vi "PH_Revolver-GUI_6P.ProcCases.vi"(0 "i ref in":refnum<vi>, 1 "selector":string, 2 "data":i8[](array[numeric]), 3 "call cluster":T1={"Object"="", "Selector"="", "CallType"=enum."synchronous", "Async Object"="", "Async Selector"="", "Data Descriptor"="", "Data"=[], "Error #"=0, "Expire"=0}, 5 "error in":errorcluster) -> (14 "i ref out":refnum<vi>, 17 "answer cluster":T1={"Object"="", "Selector"="", "CallType"=enum."synchronous", "Async Object"="", "Async Selector"="", "Data Descriptor"="", "Data"=[], "Error #"=0, "Expire"=0}, 19 "error out":errorcluster)   [LabVIEW 2014, in "PH_Revolver-GUI_6P.lvlib"]
doc: "This method is called by a process from within the default case in the event loop. The methods of a class that are linked to events will be called from THIS method. Add your code here."
uses:
  PH_Revolver-GUI_6P.lvlib
  CS_Core/CSSystem/CoreDefs/CoreDefs.call_type.ctl
  CS_Core/BaseProcess/BaseProcess.descriptor string definition.ctl
  CS_Core/CSSystem/CoreDefs/CoreDefs.rawDataType.ctl
  PH_Revolver-GUI_6P.Position.ctl
  CS_Core/CSSystem/CoreLib/CoreLib.string 2 byte array.vi
  CS_Core/CSSystem/CoreLib/CoreLib.byte array 2 short.vi
  CS_Core/BaseProcess/BaseProcess.lvlib
  CS_Core/CSSystem/CoreLib/CoreLib.lvlib
  CS_Core/CAEObj/CAEObj.lvlib
  PH_Basics/PH_PSDBWriter/PH_PSDBWriter.lvlib
  PH_Basics/PH_Stepmotor_BaseClass/PH_Stepmotor_BaseClass.lvlib
  PH_Basics/PH_AxisGUI_BaseClass/PH_AxisGUI_BaseClass.lvlib
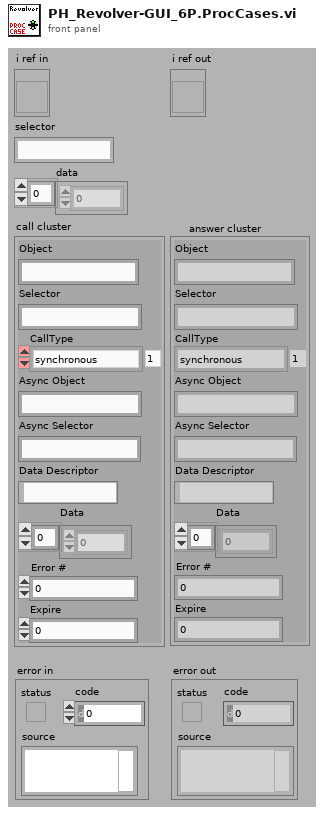
[diagram p1: front panel]
types:
  T1 = typedef "CoreDefs.call_type.ctl" = cluster{"Object":string, "Selector":string, "CallType":enum16{"simple", "synchronous", "asynchronous"}, "Async Object":string, "Async Selector":string, "Data Descriptor":T2, "Data":T3, "Error #":i32, "Expire":u32}
  T2 = typedef "BaseProcess.lvlib/BaseProcess.descriptor string definition.ctl" = string
  T3 = typedef "CoreDefs.rawDataType.ctl" = i8[]
  T4 = typedef "PH_PSDBWriter.lvlib/PH_PSDBWriter.PHELIX-Subsystems.ctl" = i32
  T5 = typedef "PH_Stepmotor_BaseClass.lvlib/PH_Stepmotor_BaseClass.Axis Information.ctl" = cluster{"Scaled Position":dbl, "Activity":T6}
  T6 = typedef "PH_Stepmotor_BaseClass.lvlib/PH_Stepmotor_BaseClass.Axis Activity.ctl" = enum16{"No Information", "stopped", "running", "Failure", "Alarm", "stopped at backward ES", "stopped at foreward ES"}
  T7 = typedef "PH_Revolver-GUI_6P.lvlib/PH_Revolver-GUI_6P.Position.ctl" = u16
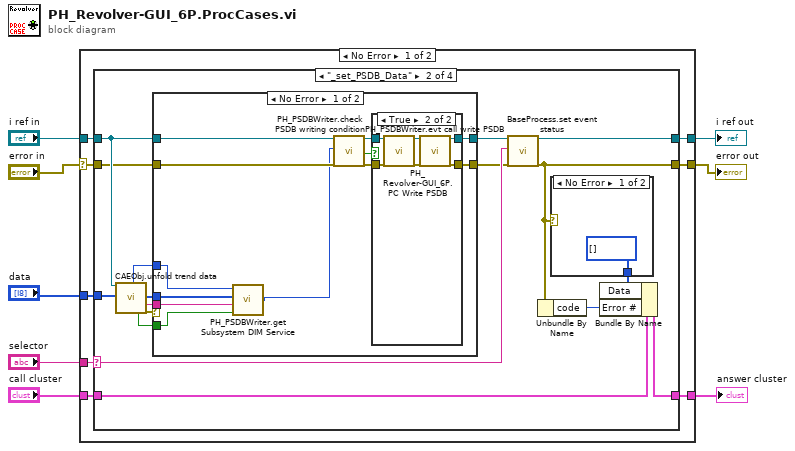
[diagram p0: block diagram]
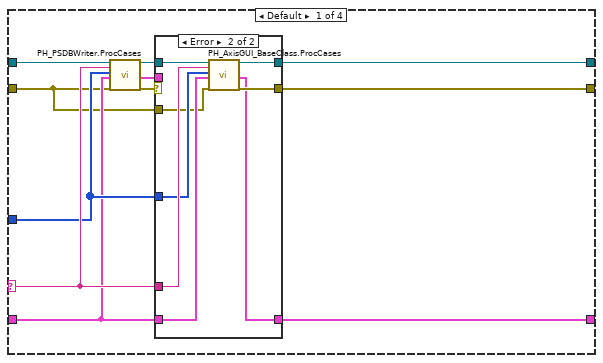
[diagram p2: hidden frame]
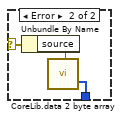
[diagram p6: hidden frame]
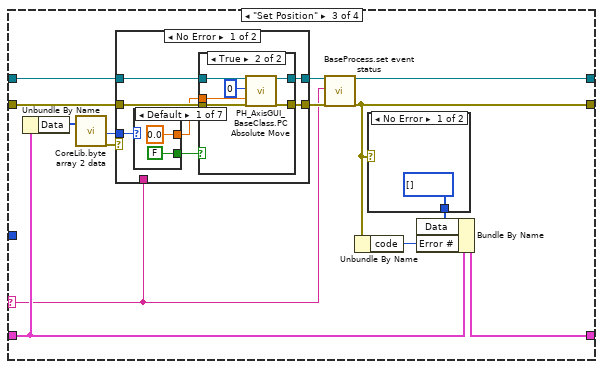
[diagram p7: hidden frame]
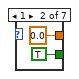
[diagram p9: hidden frame]
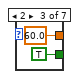
[diagram p10: hidden frame]
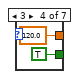
[diagram p11: hidden frame]
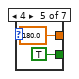
[diagram p12: hidden frame]
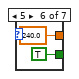
[diagram p13: hidden frame]
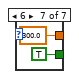
[diagram p14: hidden frame]
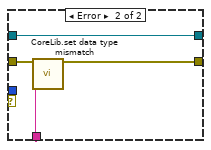
[diagram p15: hidden frame]
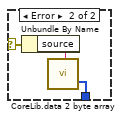
[diagram p16: hidden frame]
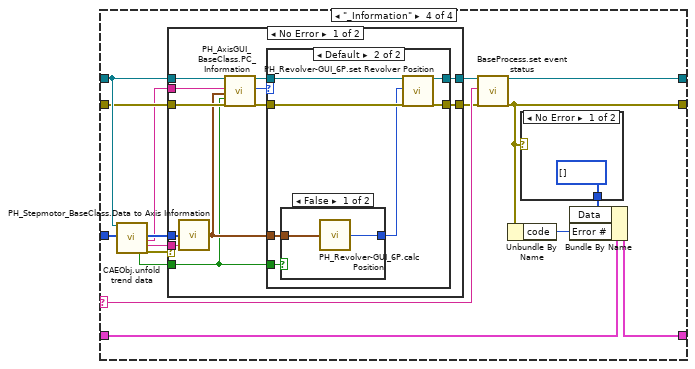
[diagram p17: hidden frame]
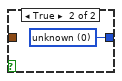
[diagram p19: hidden frame]
diagram:
  n1 = case shown="No Error" "error in" {
    selector: "error in" -> [w9 w181]
    tunnel: "selector" -> [w16 _]
    tunnel: [w15 w180] -> w7
    tunnel: "call cluster" -> [w14 w180]
    tunnel: "i ref in" -> [w13 w182]
    tunnel: [w12 w182] -> w4
    tunnel: [w11 w181] -> w3
    tunnel: "data" -> [w10 _]
    frame No Error {
      n2 = case shown="\"_set_PSDB_Data\"" w16 {
        selector: w16 -> [w22 w49 w82 w146]
        tunnel: w13 -> [w27 w43 w87 w138]
        tunnel: [w24 w52 w93 w145] -> w12
        tunnel: w14 -> [w20 w54 w86 w148]
        tunnel: [w19 w50 w91 w143] -> w15
        tunnel: w9 -> [w17 w40 w85 w136]
        tunnel: [w26 w53 w94 w147] -> w11
        tunnel: w10 -> [w21 w39 _ w134]
        frame Default {
          n3 = call "PH_PSDBWriter.ProcCases.vi"("i ref in"=w27, "selector"=w22, "Data"=w21, "call cluster"=w20, "error in"=w17) -> ("i ref out"=w25:refnum<vi>, "answer cluster"=w18:T1, "error out"=w23:errorcluster)  [unwired: 12 in]
          n4 = case shown="Error" w23 {
            selector: w23 -> [w29 _]
            tunnel: [w29 w38] -> w26
            tunnel: w25 -> [w30 w37]
            tunnel: [w30 w36] -> w24
            tunnel: w22 -> [_ w35]
            tunnel: w21 -> [_ w34]
            tunnel: w20 -> [_ w33]
            tunnel: [w28 w32] -> w19
            tunnel: w18 -> [w28 _]
            tunnel: w17 -> [_ w31]
            frame No Error {
            }
            frame Error {
              n5 = call "PH_AxisGUI_BaseClass.ProcCases.vi"("i ref in"=w37, "selector"=w35, "data"=w34, "call cluster"=w33, "error in"=w31) -> ("i ref out"=w36:refnum<vi>, "answer cluster"=w32:T1, "error out"=w38:errorcluster)  [unwired: 12 in]
            }
          }
        }
        frame "_set_PSDB_Data" {
          n6 = call "CAEObj.unfold trend data.vi"("i ref in"=w43, "raw trend data"=w39) -> ("quality"=w48:i32, "no link"=w45:bool, "data"=w47:i8[], "typeDescriptor"=w46:string, "error out"=w44:errorcluster)  [unwired: 9 in, 4 out]
          n7 = case shown="No Error" w44 {
            tunnel: w40 -> [w67 w77]
            tunnel: [w66 w76] -> w42
            tunnel: [w65 w77] -> w41
            tunnel: w43 -> [w63 w76]
            tunnel: w45 -> [w57 _]
            tunnel: w46 -> [w59 _]
            tunnel: w47 -> [w60 _]
            tunnel: w48 -> [w58 _]
            frame No Error {
              n8 = call "PH_PSDBWriter.get Subsystem DIM Service.vi"("no link"=w57, "typeDescriptor"=w59, "data"=w60, "quality"=w58) -> ("PHELIX Subsystems"=w56:T4)
              n9 = call "PH_PSDBWriter.check PSDB writing condition.vi"("i ref in"=w63, "wanted Subsystem"=w56, "error IO"=w67) -> ("i ref out"=w62:refnum<vi>, "write PSDB?"=w61:bool, "error out"=w64:errorcluster)  [unwired: 14 in]
              n10 = case shown="True" w61 {
                tunnel: w64 -> [w68 w75]
                tunnel: [w69 w72] -> w66
                tunnel: [w68 w70] -> w65
                tunnel: w62 -> [w69 w74]
                frame False {
                }
                frame True {
                  n11 = call "PH_Revolver-GUI_6P.PC Write PSDB.vi"("i ref in"=w74, "error IO"=w75) -> ("i ref out"=w73:refnum<vi>, "error out"=w71:errorcluster)  [unwired: 16 in]
                  n12 = call "PH_PSDBWriter.evt call write PSDB.vi"("i ref in"=w73, "error in (no error)"=w71) -> ("i ref out"=w72:refnum<vi>, "error out"=w70:errorcluster)  [unwired: 16 in]
                }
              }
            }
            frame Error {
            }
          }
          n13 = call "BaseProcess.set event status.vi"("i ref in"=w42, "EventStatus"=w49, "error in (no error)"=w41) -> ("i ref out"=w52:refnum<vi>, "error out"=w53:errorcluster)  [unwired: 14 in, 1 out]
          n14 = Unbundle By Name(w53) -> ("code"=w55:i32)
          n15 = case shown="No Error" w53 {
            selector: w53 -> [_ w81]
            tunnel: [T3 [] ("byteArray out") w79] -> w51
            frame No Error {
            }
            frame Error {
              n16 = Unbundle By Name(w81) -> ("source"=w80:string)
              n17 = call-poly "CoreLib.data 2 byte array.vi"("string"=w80) -> ("byteArray out"=w79:T3)  [unwired: 18 in]
            }
          }
          n18 = Bundle By Name(cluster=w54, "Data"=w51, "Error #"=w55) -> (w50:T1)
        }
        frame "Set Position" {
          n19 = Unbundle By Name(w86) -> ("Data"=w90:T3)
          n20 = call-poly "CoreLib.byte array 2 data.vi"("byteArray"=w90) -> ("i16"=w88:i16, "error out"=w89:errorcluster)  [unwired: 16 in, 1 out]
          n21 = case shown="No Error" w89 {
            tunnel: [w98 w128] -> w84
            tunnel: w87 -> [w99 w128]
            tunnel: w85 -> [w101 w127]
            tunnel: [w100 w126] -> w83
            tunnel: w82 -> [_ w125]
            tunnel: w88 -> [w102 _]
            frame No Error {
              n22 = case shown="Default" w102 {
                tunnel: [0.0 0.0 60.0 120.0 180.0 240.0 300.0] -> w97
                tunnel: [FALSE TRUE TRUE TRUE TRUE TRUE TRUE] -> w96
                frame Default {
                }
                frame 1 {
                }
                frame 2 {
                }
                frame 3 {
                }
                frame 4 {
                }
                frame 5 {
                }
                frame 6 {
                }
              }
              n23 = case shown="True" w96 {
                tunnel: w101 -> [w103 w110]
                tunnel: [w103 w109] -> w100
                tunnel: w99 -> [w104 w108]
                tunnel: [w104 w107] -> w98
                tunnel: w97 -> [_ w106]
                frame False {
                }
                frame True {
                  n24 = call "PH_AxisGUI_BaseClass.PC Absolute Move.vi"("i ref in"=w108, "Axis"=0, "Position [Units]"=w106, "error in"=w110) -> ("i ref out"=w107:refnum<vi>, "error out"=w109:errorcluster)  [unwired: 14 in]
                }
              }
            }
            frame Error {
              n25 = call "CoreLib.set data type mismatch.vi"("error in (no error)"=w127, "error source"=w125) -> ("error out"=w126:errorcluster)  [unwired: 17 in]
            }
          }
          n26 = call "BaseProcess.set event status.vi"("i ref in"=w84, "EventStatus"=w82, "error in (no error)"=w83) -> ("i ref out"=w93:refnum<vi>, "error out"=w94:errorcluster)  [unwired: 14 in, 1 out]
          n27 = Unbundle By Name(w94) -> ("code"=w95:i32)
          n28 = case shown="No Error" w94 {
            selector: w94 -> [_ w132]
            tunnel: [T3 [] ("byteArray out") w130] -> w92
            frame No Error {
            }
            frame Error {
              n29 = Unbundle By Name(w132) -> ("source"=w131:string)
              n30 = call-poly "CoreLib.data 2 byte array.vi"("string"=w131) -> ("byteArray out"=w130:T3)  [unwired: 18 in]
            }
          }
          n31 = Bundle By Name(cluster=w86, "Data"=w92, "Error #"=w95) -> (w91:T1)
        }
        frame "_Information" {
          n32 = call "CAEObj.unfold trend data.vi"("i ref in"=w138, "raw trend data"=w134) -> ("no link"=w139:bool, "data"=w142:i8[], "serviceName"=w133:string, "typeDescriptor"=w140:string, "error out"=w141:errorcluster)  [unwired: 9 in, 4 out]
          n33 = case shown="No Error" w141 {
            tunnel: w142 -> [w161 _]
            tunnel: w138 -> [w159 w175]
            tunnel: [w156 w175] -> w137
            tunnel: w136 -> [w158 w174]
            tunnel: w139 -> [w150 _]
            tunnel: w140 -> [w160 _]
            tunnel: [w154 w174] -> w135
            tunnel: w133 -> [w153 _]
            frame No Error {
              n34 = call "PH_Stepmotor_BaseClass.Data to Axis Information.vi"("data"=w161, "Type Descriptor"=w160) -> ("Axis Information"=w151:T5)
              n35 = call "PH_AxisGUI_BaseClass.PC_Information.vi"("i ref in"=w159, "Service Name"=w153, "Axis Information"=w151, "no link"=w150, "error in"=w158) -> ("i ref out"=w157:refnum<vi>, "Axis"=w152:i32, "error out"=w155:errorcluster)  [unwired: 12 in]
              n36 = case shown="Default" w152 {
                tunnel: w157 -> [w163 w170]
                tunnel: [w163 w169] -> w156
                tunnel: w155 -> [w162 w168]
                tunnel: [w162 w167] -> w154
                tunnel: w151 -> [_ w166]
                tunnel: w150 -> [_ w164]
                frame -1 {
                }
                frame Default {
                  n37 = case shown="False" w164 {
                    tunnel: w166 -> [w172 _]
                    tunnel: [w171 w173] -> w165
                    frame False {
                      n38 = call "PH_Revolver-GUI_6P.calc Position.vi"("Axis Information"=w172) -> ("Revolver Position"=w171:T7)
                    }
                    frame True {
                      w173 = T7 0 items=["unknown", "Position 0", "Position 60", "Position 120", "Position 180", "Position 240", "Position 300", "moving"] ("Revolver Position")
                    }
                  }
                  n39 = call "PH_Revolver-GUI_6P.set Revolver Position.vi"("VI in"=w170, "Revolver Position"=w165, "error in (no error)"=w168) -> ("VI out"=w169:refnum<vi>, "error out"=w167:errorcluster)  [unwired: 15 in]
                }
              }
            }
            frame Error {
            }
          }
          n40 = call "BaseProcess.set event status.vi"("i ref in"=w137, "EventStatus"=w146, "error in (no error)"=w135) -> ("i ref out"=w145:refnum<vi>, "error out"=w147:errorcluster)  [unwired: 14 in, 1 out]
          n41 = Unbundle By Name(w147) -> ("code"=w149:i32)
          n42 = case shown="No Error" w147 {
            selector: w147 -> [_ w179]
            tunnel: [T3 [] ("byteArray out") w177] -> w144
            frame No Error {
            }
            frame Error {
              n43 = Unbundle By Name(w179) -> ("source"=w178:string)
              n44 = call-poly "CoreLib.data 2 byte array.vi"("string"=w178) -> ("byteArray out"=w177:T3)  [unwired: 18 in]
            }
          }
          n45 = Bundle By Name(cluster=w148, "Data"=w144, "Error #"=w149) -> (w143:T1)
        }
      }
    }
    frame Error {
    }
  }
  "answer cluster" <- w7
  "i ref out" <- w4
  "error out" <- w3
